vi "HAL_Configure RF.vi"(8 "error in":errorcluster, 9 "Level":dbl, 10 "Frequency (Hz)":dbl, 11 "Handle In":T1) -> (0 "error out":errorcluster, 3 "Handle Out":T1)   [LabVIEW 2015]
uses:
  Handle.ctl
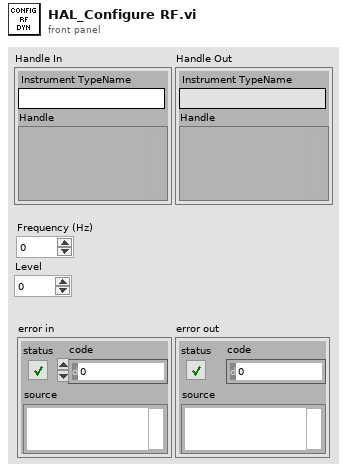
[diagram p1: front panel]
types:
  T1 = typedef "Handle.ctl" = cluster{"Instrument TypeName":string, "Handle":variant}
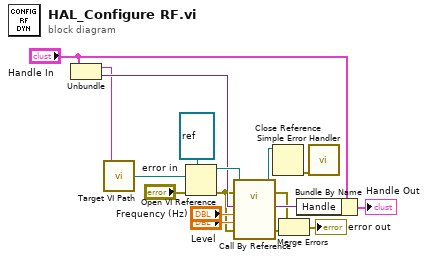
[diagram p0: block diagram]
diagram:
  n1 = Unbundle("Handle In") -> ("Instrument TypeName"=w6:string, "Handle"=w15:variant)
  n2 = call "Target VI Path.vi"("Instrument Name"=w6) -> ("Path to VI"=w7:path)
  n3 = Open VI Reference(type specifier VI Refnum (for type only)=refnum<vi> refnum, vi path=w7, error in (no error)="error in") -> (vi reference=w16:refnum<vi>, error out=w4:errorcluster)  [unwired: 3 in]
  n4 = call-by-ref "?"(reference=w16, error in=w4, "error in"=w4, "Level"="Level", "Frequency (Hz)"="Frequency (Hz)", "Handle In"=w15) -> (reference out=w2:refnum<vi>, error out=w3:errorcluster, 0:"error out"=w11:errorcluster, "Handle Out"=w13:variant)  [unwired: 6 in]
  n5 = Close Reference(reference=w2) -> (error out=w1:errorcluster)  [unwired: 1 in]
  n6 = Merge Errors(w3, w11) -> (→"error out":errorcluster)
  n7 = Bundle By Name(cluster="Handle In", "Handle"=w13) -> (→"Handle Out":T1)
  n8 = call <vilib>:"Simple Error Handler.vi"("error in (no error)"=w1) -> ()  [unwired: 4 in, 5 out]
